vi "SERIAL_OpenInternal.vi"(11 "Serial Port (MXP)":T2=enum."MXP TTL") -> (0 "error out":errorcluster, 1 "Opened":bool, 3 "SerialPortRef":T1)   [LabVIEW 2014, in "navX-MXP IMU.lvlib"]
uses:
  navX-MXP IMU.lvlib
  NI WPI/WPI_SerialPort_USB.ctl
  <vilib>/Rock Robotics/WPI/SerialPort/WPI_SerialPortRef.ctl
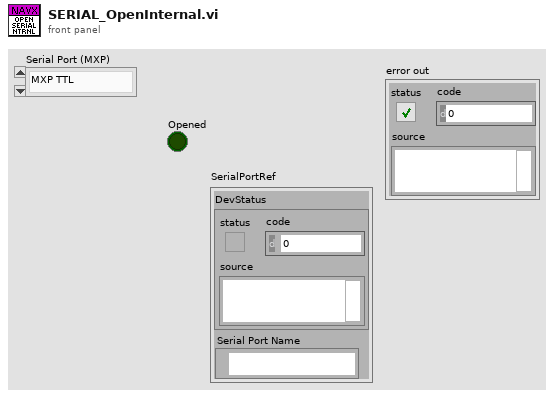
[diagram p1: front panel]
types:
  T1 = typedef "WPI_SerialPortRef.ctl" = cluster{"DevStatus":errorcluster, "Serial Port Name":refnum<visa-resource-name>}
  T2 = typedef "navX-MXP IMU.lvlib/WPI_SerialPort_USB.ctl" = enum16{"Onboard RS-232", "MXP TTL", "USB"}
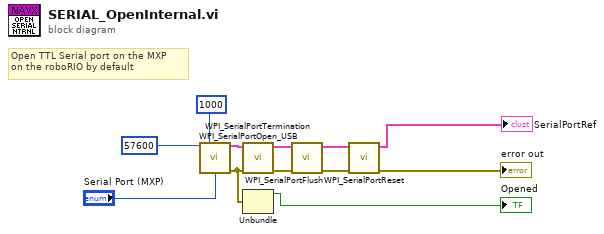
[diagram p0: block diagram]
diagram:
  # "Open TTL Serial port on the MXP \non the roboRIO by default"
  n1 = call "WPI_SerialPortOpen_USB.vi"("Baud Rate"=u32 57600, "Timeout Value (ms)"=u32 1000, "Serial Port"="Serial Port (MXP)") -> ("SerialPortRef"=w7:T1, "error out"=w4:errorcluster)  [unwired: 11 in]
  n2 = call <vilib>:"WPI_SerialPortTermination.vi"("error in (no error)"=w4, "SerialPortRef"=w7) -> ("error out"=w12:errorcluster, "SerialPortRef"=w11:T1)  [unwired: 8 in]
  n3 = Unbundle(w4) -> ("status"=→"Opened":bool)  [unwired: 2 out]
  n4 = call <vilib>:"WPI_SerialPortFlush.vi"("error in (no error)"=w12, "SerialPortRef"=w11) -> ("error out"=w10:errorcluster, "SerialPortRef"=w9:T1)  [unwired: 8 in]
  n5 = call <vilib>:"WPI_SerialPortReset.vi"("error in (no error)"=w10, "SerialPortRef"=w9) -> ("error out"=→"error out":errorcluster, "SerialPortRef"=→"SerialPortRef":T1)  [unwired: 8 in]
